vi "Destroy to SSH.vi"(8 "Error In":errorcluster, 11 "Identity":refnum<class "Agent Identity.lvclass">) -> (0 "Error Out":errorcluster, 3 "SSH":refnum<class "SSH.lvclass">)   [LabVIEW 2021, in "Field_RnD_Services_LIBSSH2_Toolkit.lvlib" / "Agent Identity.lvclass"]
doc: "Destroys this Agent Identity object and returns the SSH context used to originally create it."
uses:
  220524-VNA RP FLAT.llb/Agent Identity.lvclass
  220524-VNA RP FLAT.llb/SSH.lvclass
  220524-VNA RP FLAT.llb/Agent Identity.lvclass/Agent Identity.ctl
  220524-VNA RP FLAT.llb/Field_RnD_Services_LIBSSH2_Toolkit.lvlib
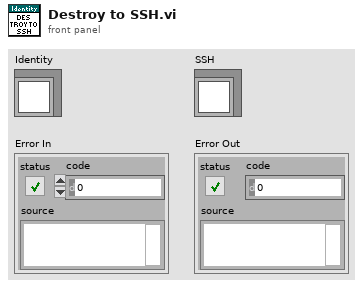
[diagram p1: front panel]
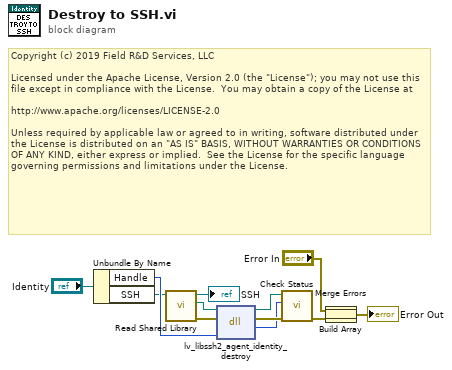
[diagram p0: block diagram]
diagram:
  # "Copyright (c) 2019 Field R&D Services, LLC\n\nLicensed under the Apache License, Version 2.0 (the \"License\"); you may not use this file except in compliance with the License.  You may obtain a copy of the License at\n\nhttp://www.apache.org/licenses/LICENSE-2.0\n\nUnless required by applicable law or agreed to in writing, software distributed under the License is distributed on an \"AS IS\" BASIS, WITHOUT WARRANTIES OR CONDITIONS OF ANY KIND, either express or implied.  See the License for the specific language governing permissions and limitations under the License."
  n1 = Unbundle By Name("Identity") -> ("Handle"=w11:u64, "SSH"=w6:refnum<class "SSH.lvclass">)
  n2 = call "Read Shared Library.vi"("SSH In"=w6) -> ("Error Out"=w5:errorcluster, "libssh2lv Shared Library"=w4:path, "SSH Out"=→"SSH":refnum<class "SSH.lvclass">)  [unwired: 8 in]
  n3 = dll-call lib="libssh2lv.*" fn="lv_libssh2_agent_identity_destroy"(path in=w4, error in=w5, "handle"=w11) -> (path out=w9:path, error out=w10:errorcluster, "status"=w8:i32)  [unwired: 2 in]
  n4 = call "Check Status.vi"("Error In"=w10, "Status"=w8, "libssh2lv Shared Library In"=w9) -> ("Error Out"=w7:errorcluster)  [unwired: 7 in, 1 out]
  n5 = Build Array("Error In", w7) -> (w1:errorcluster[])
  n6 = Merge Errors(w1) -> (→"Error Out":errorcluster)
